vi "DSF.Engine.Memory.Cache.Plugin.Get Largest Count.All Types.vi"(8 "error in (no error)":errorcluster, 10 "Data Type Counts in":T1 {"U64" format="%d elements"; "U32" format="%d elements"; "U16" format="%d elements"; "U8" format="%d elements"; "I64" format="%d elements"; "I32" format="%d elements"; "I16" format="%d elements"; "I8" format="%d elements"; "DBL" format="%d elements"; "SGL" format="%d elements"; "Bool" format="%d elements"}, 11 "Plugin Cache in":refnum<class "DSF.Engine.Memory.Cache.Plugin.lvclass">) -> (0 "error out":errorcluster, 2 "Data Type Counts out":T1 {"U64" format="%d elements"; "U32" format="%d elements"; "U16" format="%d elements"; "U8" format="%d elements"; "I64" format="%d elements"; "I32" format="%d elements"; "I16" format="%d elements"; "I8" format="%d elements"; "DBL" format="%d elements"; "SGL" format="%d elements"; "Bool" format="%d elements"}, 3 "Plugin Cache out":refnum<class "DSF.Engine.Memory.Cache.Plugin.lvclass">)   [LabVIEW 2016, in "DSF.Engine.lvlib" / "DSF.Engine.Memory.Cache.Plugin.lvclass"]
uses:
  DSF.Engine.Memory.Cache.Plugin.lvclass
  Shared/Typedefs/DSF.Shared.Typedefs.Data Type Counts.ctl
  DSF.Engine.Memory.Cache.Plugin.lvclass/DSF.Engine.Memory.Cache.Plugin.ctl
  DSF.Engine.Memory.Cache.Transfer Group.lvclass
  DSF.Shared.lvlib
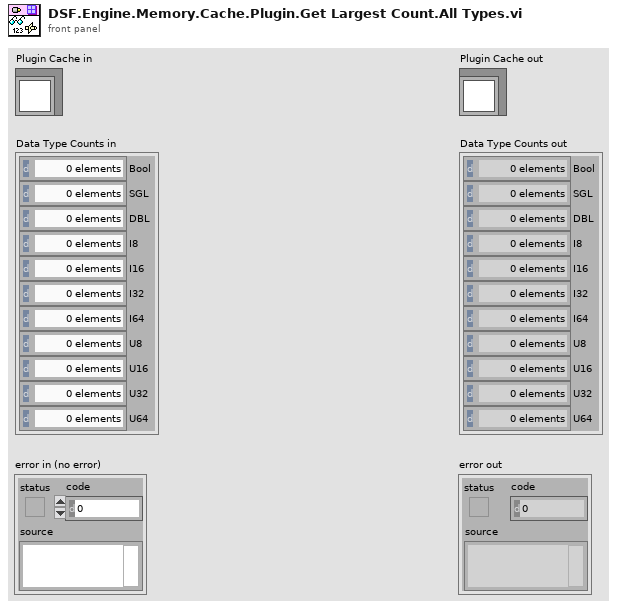
[diagram p1: front panel]
types:
  T1 = typedef "DSF.Shared.lvlib/DSF.Shared.Typedefs.Data Type Counts.ctl" = cluster{"Bool":u64, "SGL":u64, "DBL":u64, "I8":u64, "I16":u64, "I32":u64, "I64":u64, "U8":u64, "U16":u64, "U32":u64, "U64":u64}
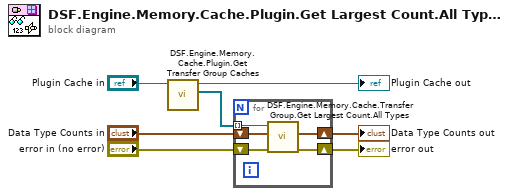
[diagram p0: block diagram]
diagram:
  n1 = call "DSF.Engine.Memory.Cache.Plugin.Get Transfer Group Caches.vi"("Plugin Cache in"="Plugin Cache in") -> ("Transfer Group Caches"=w6:refnum<class "DSF.Engine.Memory.Cache.Transfer Group.lvclass">[], "Plugin Cache out"=→"Plugin Cache out":refnum<class "DSF.Engine.Memory.Cache.Plugin.lvclass">)  [unwired: 9 in]
  n2 = for {
    shift-right: [w12] -> w2
    shift-left: "Data Type Counts in" -> [w11]
    tunnel: w6 -> [w10] mode=indexing
    shift-right: [w8] -> w4
    shift-left: "error in (no error)" -> [w9]
    n3 = call "DSF.Engine.Memory.Cache.Transfer Group.Get Largest Count.All Types.vi"("error in (no error)"=w9, "Data Type Counts in"=w11, "Transfer Group Cache in"=w10) -> ("error out"=w8:errorcluster, "Data Type Counts out"=w12:T1)  [unwired: 6 in, 1 out]
  }
  "error out" <- w4
  "Data Type Counts out" <- w2
